vi "act_4-conv_C_F.vi"() -> ()   [LabVIEW 2010]
panel:
  out "DEG F":dbl
  in  "DEG C":dbl
  out "deg F":dbl
  in  "deg C":dbl
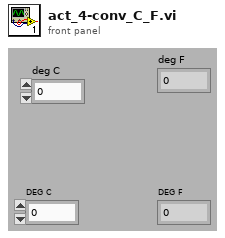
[diagram p1: front panel]
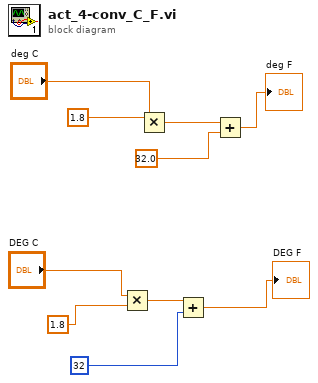
[diagram p0: block diagram]
diagram:
  n1 = Multiply(x="DEG C", y=1.8) -> (x*y=w4:dbl)
  n2 = Multiply(x=1.8, y="deg C") -> (x*y=w6:dbl)
  n3 = Add(x=w4, y=32) -> (x+y=→"DEG F":dbl)
  n4 = Add(x=w6, y=32.0) -> (x+y=→"deg F":dbl)
